vi "Make Waterfall.vi"(9 "Append":bool, 10 "Delta":dbl=1.0, 11 "Chart":dbl[](array[numeric])) -> (3 "Graph":dbl[][](array[numeric]))   [LabVIEW 2019]
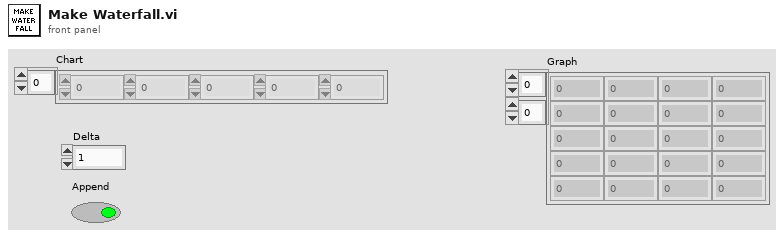
[diagram p1: front panel]
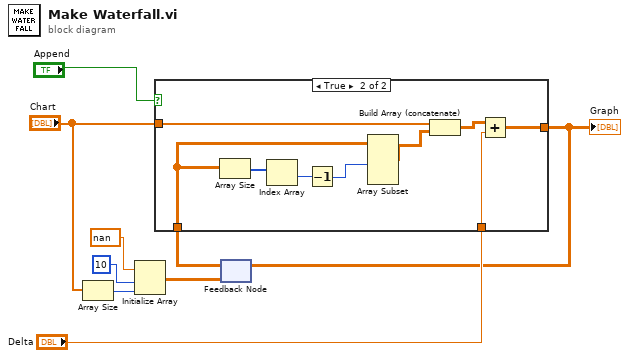
[diagram p0: block diagram]
diagram:
  n1 = Array Size(array="Chart") -> (size(s)=w7:i32)
  n2 = Initialize Array(nan ("element"), 10, w7) -> (w4:dbl[][])
  n3 = feedback #1(w4) -> (w9:dbl[][])
  n4 = case shown="True" "Append" {
    tunnel: w9 -> [w10 w19]
    tunnel: "Chart" -> [_ w15]
    tunnel: "Delta" -> [_ w14]
    tunnel: [w10 w11] -> w2
    frame False {
    }
    frame True {
      n5 = Array Size(array=w19) -> (size(s)=w18:i32[])
      n6 = Index Array(array=w18) -> (element=w17:i32)  [unwired: 1 in]
      n7 = Decrement(x=w17) -> (x-1=w16:i32)
      n8 = Array Subset(array=w19, length (row)=w16) -> (w13:dbl[][])  [unwired: 3 in]
      n9 = Build Array (concatenate)(w15, w13) -> (w12:dbl[][])
      n10 = Add(x=w12, y=w14) -> (x+y=w11:dbl[][])
    }
  }
  "Graph" <- w2
  n11 = feedback-in #1(w2) -> ()
